vi "SaveSeqToXML.vi"(8 "error in (no error)":errorcluster, 11 "TestSeqClass in":refnum<class "TestSeqClass.lvclass">) -> (0 "error out":errorcluster, 3 "TestSeqClass out":refnum<class "TestSeqClass.lvclass">)   [LabVIEW 2017, in "TestSeqClass.lvclass"]
uses:
  TestSeqClass.lvclass
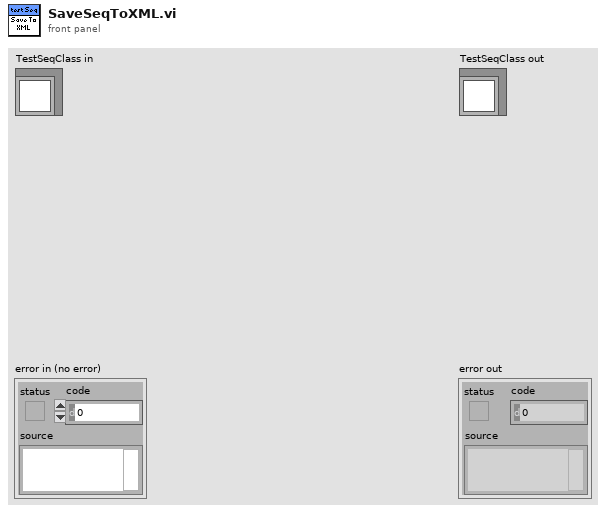
[diagram p1: front panel]
types:
  T1 = enum16{"open", "open or create", "create or replace", "create", "open (read only)"}
  T2 = typedef "TestSeqType.ctl" = refnum<class "TestMeasureStep.lvclass">[]
  T3 = typedef "TestTypeSelect.ctl" = enum16{"Calibration", "Testing"}
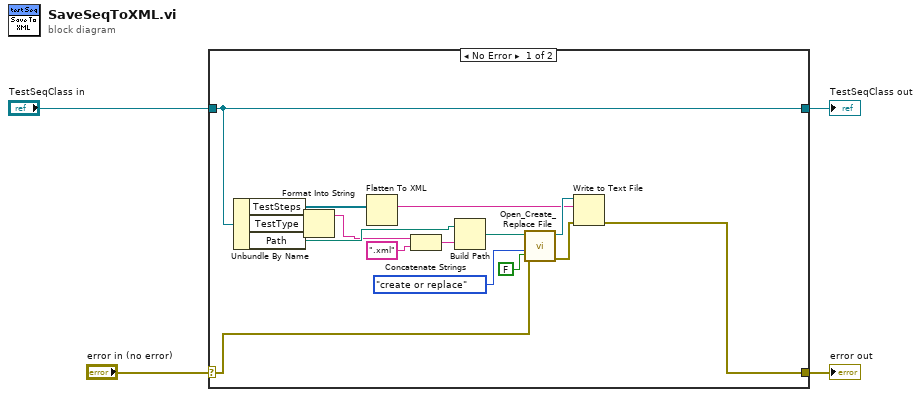
[diagram p0: block diagram]
diagram:
  n1 = case shown="No Error" "error in (no error)" {
    selector: "error in (no error)" -> [w12 w21]
    tunnel: [w11 w21] -> w3
    tunnel: [w19 w20] -> w1
    tunnel: "TestSeqClass in" -> [w19 w20]
    frame No Error {
      n2 = Unbundle By Name(w19) -> ("TestSteps"=w14:T2, "TestType"=w6:T3, "Path"=w8:path)
      n3 = Format Into String(w6) -> (resulting string=w5:string)  [unwired: 3 in, 1 out]
      n4 = Flatten To XML(anything=w14) -> (xml string=w13:string)
      n5 = Concatenate Strings(w5, ".xml" ("string")) -> (w9:string)
      n6 = Build Path(base path=w8, name or relative path=w9) -> (appended path=w7:path)
      n7 = call <vilib>:"Open_Create_Replace File.vi"("advisory dialog? (display:T)"=FALSE, "error in (no error)"=w12, "function (open:0)"=T1."create or replace", "file path"=w7) -> ("error out"=w16:errorcluster, "refnum"=w15:refnum<file>)  [unwired: 3 in, 3 out]
      n8 = Write to Text File(file (use dialog)=w15, text=w13, error in=w16) -> (error out=w11:errorcluster)  [unwired: 1 in, 2 out]
    }
    frame Error {
    }
  }
  "error out" <- w3
  "TestSeqClass out" <- w1
